vi "BigIntArrayMultiply.vi"(1 "b":u64[](array[numeric]), 2 "a":u64[](array[numeric])) -> (0 "a * b":u64[](array[numeric]))   [LabVIEW 2023]
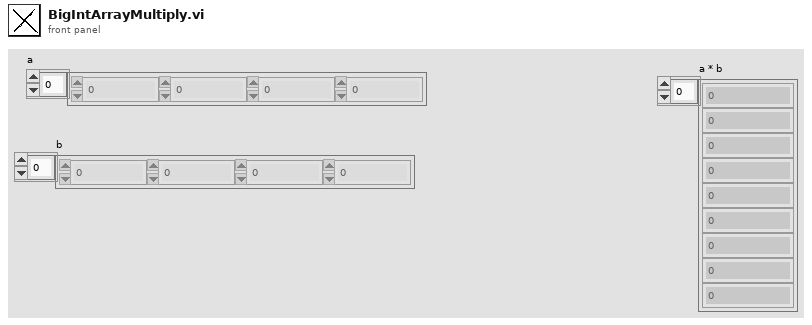
[diagram p1: front panel]
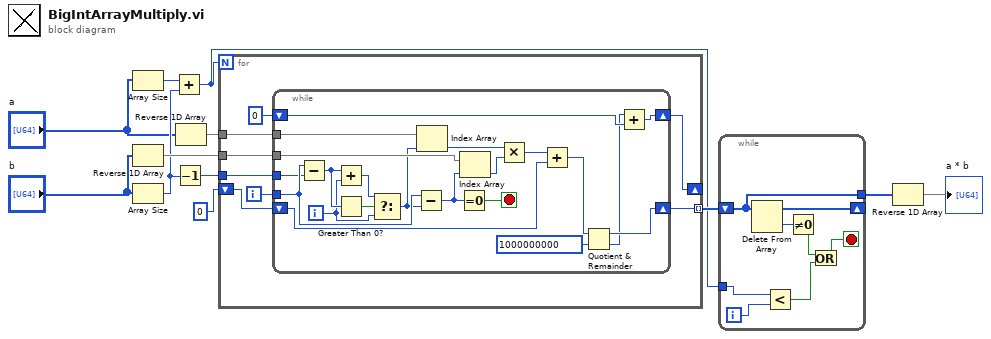
[diagram p0: block diagram]
diagram:
  n1 = Array Size(array="a") -> (size(s)=w12:i32)
  n2 = Reverse 1D Array(array="b") -> (reversed array=w10:u64[])
  n3 = Array Size(array="b") -> (size(s)=w6:i32)
  n4 = Add(x=w12, y=w6) -> (x+y=w1:i32)
  n5 = Decrement(x=w6) -> (x-1=w5:i32)
  n6 = Reverse 1D Array(array="a") -> (reversed array=w11:u64[])
  n7 = for {
    N: w1 -> [_]
    tunnel: w11 -> [w19]
    tunnel: w10 -> [w18]
    tunnel: [w16] -> w8 mode=indexing
    shift-right: [w15] -> _
    shift-left: u64 0 -> [w14]
    tunnel: w5 -> [w13]
    i -> [w20]
    n8 = while {
      tunnel: w20 -> [w27]
      tunnel: w19 -> [w41]
      tunnel: w18 -> [w40]
      shift-right: [w29] -> w16
      shift-left: w14 -> [w36]
      shift-right: [w32] -> w15
      shift-left: u64 0 -> [w33]
      tunnel: w13 -> [w26]
      i -> [w22]
      stop <- w30 stop-if-true
      n9 = Subtract(x=w27, y=w26) -> (x-y=w23:i32)
      n10 = Add(x=w23, y=w22) -> (x+y=w21:i32)
      n11 = Greater Than 0?(x=w23) -> (x > 0?=w24:bool)
      n12 = Select(t=w21, s=w24, f=w22) -> (s? t:f=w25:i32)
      n13 = Subtract(x=w27, y=w25) -> (x-y=w31:i32)
      n14 = Index Array(array=w41, index=w25) -> (element=w39:u64)
      n15 = Equal To 0?(x=w31) -> (x = 0?=w30:bool)
      n16 = Index Array(array=w40, index=w31) -> (element=w38:u64)
      n17 = Multiply(x=w39, y=w38) -> (x*y=w35:u64)
      n18 = Add(x=w35, y=w36) -> (x+y=w34:u64)
      n19 = Quotient & Remainder(x=w34, y=u64 1000000000) -> (x-y*floor(x/y)=w29:u64, floor(x/y)=w28:u64)
      n20 = Add(x=w28, y=w33) -> (x+y=w32:u64)
    }
  }
  n21 = while {
    shift-right: [w49] -> _
    shift-left: w8 -> [w48]
    tunnel: [w48] -> w7
    tunnel: w1 -> [w46]
    i -> [w45]
    stop <- w42 stop-if-true
    n22 = Delete From Array(array=w48) -> (deleted portion=w47:u64, array with subset deleted=w49:u64[])  [unwired: 2 in]
    n23 = Less?(x=w46, y=w45) -> (x < y?=w43:bool)
    n24 = Not Equal To 0?(x=w47) -> (x != 0?=w44:bool)
    n25 = Or(x=w44, y=w43) -> (x .or. y?=w42:bool)
  }
  n26 = Reverse 1D Array(array=w7) -> (reversed array=→"a * b":u64[])
